vi "Clean Response.vi"(8 "error in (no error)":errorcluster, 10 "Response In":string, 11 "PID.lvclass":refnum<class "PID.lvclass">) -> (0 "error out":errorcluster, 2 "result string":string, 3 "PID.lvclass 2":refnum<class "PID.lvclass">)   [LabVIEW 2011, in "PID.lvclass"]
uses:
  PID.lvclass
  PID.lvclass/PID.ctl
panel:
  out "offset past match":i32
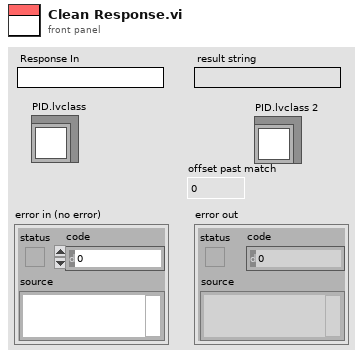
[diagram p1: front panel]
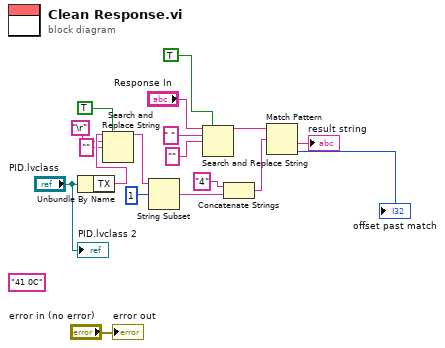
[diagram p0: block diagram]
diagram:
  (unwired) "41 0C" ("regular expression")
  n1 = Unbundle By Name("PID.lvclass") -> ("TX"=w5:string)
  n2 = Search and Replace String(replace all?=TRUE ("replace all? (F)"), input string=w5, search string="\r", replace string="" ("replace string (\"\")")) -> (result string=w4:string)  [unwired: 4 in, 3 out]
  n3 = String Subset(string=w4, offset (0)=1) -> (substring=w14:string)  [unwired: 1 in]
  n4 = Search and Replace String(replace all?=TRUE ("replace all? (F)"), input string="Response In", search string=" ", replace string="" ("replace string (\"\")")) -> (result string=w7:string)  [unwired: 4 in, 3 out]
  n5 = Concatenate Strings("4" ("string"), w14) -> (w12:string)
  n6 = Match Pattern(string=w7, regular expression=w12) -> (after substring=→"result string":string, offset past match=→"offset past match":i32)  [unwired: 1 in, 2 out]
  "PID.lvclass 2" <- "PID.lvclass"
  "error out" <- "error in (no error)"
